vi "SetParametrsOfPanels.vi"(9 "MainMenu_In":refnum<vi>, 10 "KEITHLEY 2182 & KEITHLEY 6222":refnum<vi>, 11 "OtherDivice_In":refnum<vi>) -> (1 "Main menu out":refnum<vi>, 2 "KEITHLEY 2182 & KEITHLEY 6221":refnum<vi>, 3 "Cluster out":refnum<vi>)   [LabVIEW 2013]
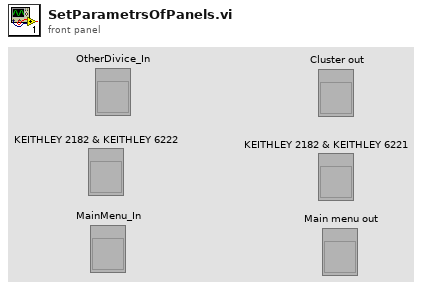
[diagram p1: front panel]
types:
  T1 = cluster{"Measurement":bool, "Save Data":bool, "LoadSetting":bool, "Save setting":bool, "Reset setting":bool, "Exit":bool}
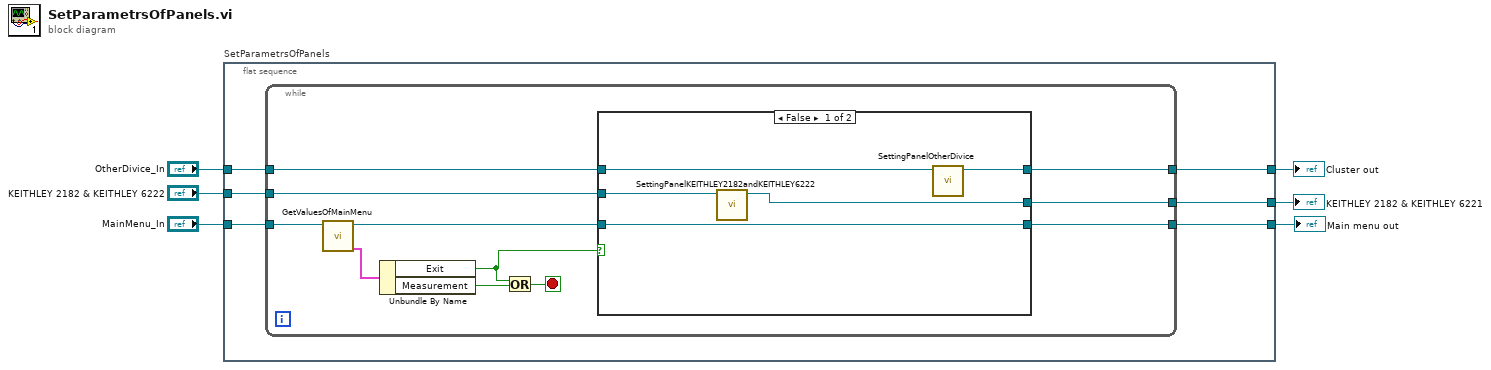
[diagram p0: block diagram]
diagram:
  n1 = flat-sequence "SetParametrsOfPanels" {
    tunnel: [w9] -> w4
    tunnel: "KEITHLEY 2182 & KEITHLEY 6222" -> [w10]
    tunnel: "MainMenu_In" -> [w8]
    tunnel: [w7] -> w3
    tunnel: [w11] -> w6
    tunnel: "OtherDivice_In" -> [w12]
    frame #0 {
      n2 = while {
        tunnel: w12 -> [w22]
        tunnel: [w23] -> w11
        tunnel: w10 -> [w20]
        tunnel: [w21] -> w9
        tunnel: w8 -> [w18]
        tunnel: [w19] -> w7
        stop <- w15 stop-if-true
        n3 = call "GetValuesOfMainMenu.vi"("MainMenu_In"=w18) -> ("ValuesOfMainMenu"=w16:T1, "MainMenu_Out"=w17:refnum<vi>)  [unwired: 9 in]
        n4 = Unbundle By Name(w16) -> ("Exit"=w14:bool, "Measurement"=w13:bool)
        n5 = Or(x=w14, y=w13) -> (x .or. y?=w15:bool)
        n6 = case shown="False" w14 {
          tunnel: [w24 w31] -> w23
          tunnel: w22 -> [w25 w31]
          tunnel: [w26 w30] -> w21
          tunnel: w20 -> [w27 w30]
          tunnel: [w28 w29] -> w19
          tunnel: w17 -> [w28 w29]
          frame False {
            n7 = call "SettingPanelKEITHLEY2182andKEITHLEY6222.vi"("KEITHLEY2182andKEITHLEY6222_In"=w27) -> ("KEITHLEY2182andKEITHLEY6222_out"=w26:refnum<vi>)  [unwired: 10 in]
            n8 = call "SettingPanelOtherDivice.vi"("OtherDivice_In"=w25) -> ("OtherDivice_Out"=w24:refnum<vi>)  [unwired: 10 in]
          }
          frame True {
            # "If Exit true, to do nothing"
          }
        }
      }
    }
  }
  "Cluster out" <- w6
  "KEITHLEY 2182 & KEITHLEY 6221" <- w4
  "Main menu out" <- w3
